vi "Get Connect Messages for Connection Lists.vi"(8 "error in (no error)":errorcluster, 10 "Communication Configuration":T3, 11 "Connection Lists for each Resource":cluster{T2[]}[](array[cluster])) -> (0 "error out":errorcluster, 3 "Messages":T1[](array[typedef]))   [LabVIEW 2017, in "Routing and Faulting Engine.lvlib"]
uses:
  Routing and Faulting Engine.lvlib
  Shared/Communication Configuration.ctl
  Shared/Connection.ctl
  Producer Message.ctl
  Includes/CDMessaging.lvlibp/Message/Abstract Message/Abstract Message.lvclass
  Includes/CDMessaging.lvlibp/Switch/Switch Connect Message/Switch Connect Message.lvclass
  C:/Users/nitest/Documents/ni-official/niveristand-routing-and-faulting-custom-device/Includes/CDMessaging.lvlibp/Message/Abstract Message/Abstract Message.lvclass
  Shared/Routing and Faulting Shared.lvlib
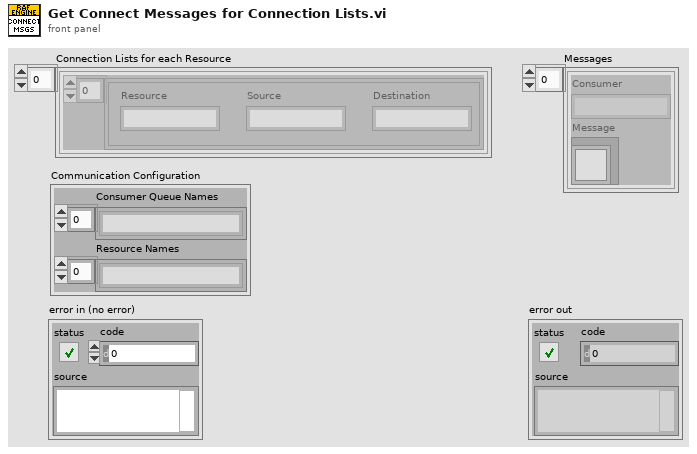
[diagram p1: front panel]
types:
  T1 = typedef "Routing and Faulting Engine.lvlib/Producer Message.ctl" = cluster{"Consumer":string, "Message":refnum<class "Abstract Message.lvclass">}
  T2 = typedef "Routing and Faulting Shared.lvlib/Connection.ctl" = cluster{"Resource":string, "Source":string, "Destination":string}
  T3 = typedef "Routing and Faulting Shared.lvlib/Communication Configuration.ctl" = cluster{"Consumer Queue Names":string[], "Resource Names":string[]}
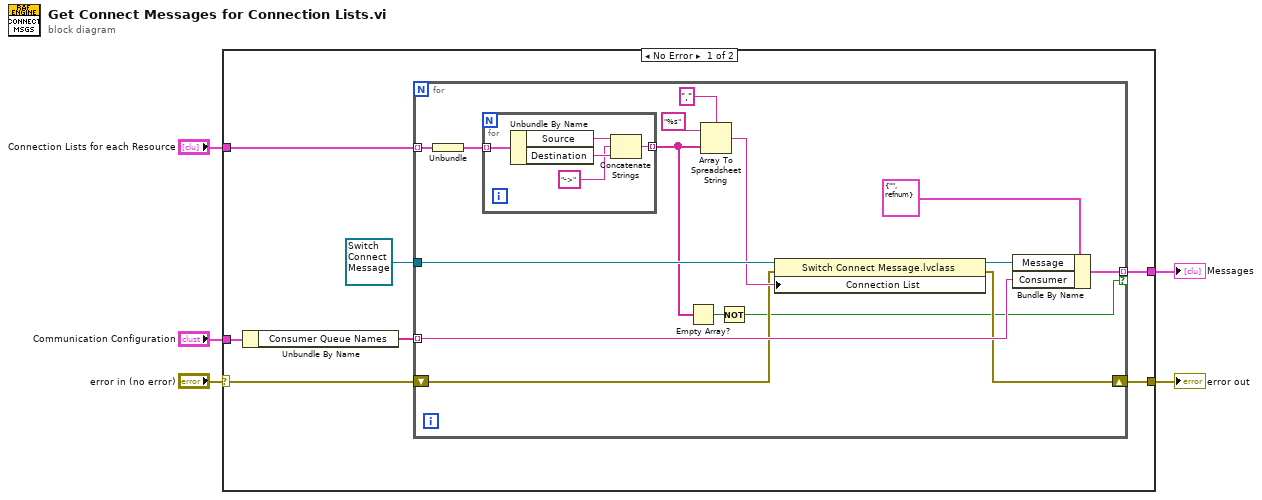
[diagram p0: block diagram]
diagram:
  n1 = case shown="No Error" "error in (no error)" {
    selector: "error in (no error)" -> [w7 w33]
    tunnel: "Communication Configuration" -> [w12 _]
    tunnel: "Connection Lists for each Resource" -> [w10 _]
    tunnel: [w9 _] -> w3
    tunnel: [w6 w33] -> w1
    frame No Error {
      n2 = Unbundle By Name(w12) -> ("Consumer Queue Names"=w11:string[])
      n3 = for {
        tunnel: w10 -> [w27] mode=indexing
        tunnel: w11 -> [w20] mode=indexing
        tunnel: refnum<class "Switch Connect Message.lvclass"> refnum ("CDMessaging.lvlibp:Switch Connect Message.lvclass") -> [w24]
        tunnel: [w19] -> w9 mode=indexing if=w13
        shift-right: [w14] -> w6
        shift-left: w7 -> [w15]
        n4 = Unbundle(w27) -> (w17:T2[])
        n5 = for {
          tunnel: w17 -> [w32] mode=indexing
          tunnel: [w28] -> w16 mode=indexing
          n6 = Unbundle By Name(w32) -> ("Source"=w31:string, "Destination"=w30:string)
          n7 = Concatenate Strings(w31, "->" ("string"), w30) -> (w28:string)
        }
        n8 = Empty Array?(array=w16) -> (empty?=w18:bool)
        n9 = Array To Spreadsheet String(delimiter (Tab)=",", array=w16, 3:"%s" ("format string")) -> (spreadsheet string=w23:string)
        n10 = Not(x=w18) -> (.not. x?=w13:bool)
        n11 = property class="Switch Connect Message.lvclass"(reference=w24, error in=w15, "Connection List"=w23) -> (reference out=w21:refnum<class "Switch Connect Message.lvclass">, error out=w14:errorcluster)
        n12 = Bundle By Name(cluster=T1 {"Consumer"="", "Message"=refnum} ("Producer Message"), "Message"=w21, "Consumer"=w20) -> (w19:T1)
      }
    }
    frame Error {
    }
  }
  "Messages" <- w3
  "error out" <- w1
